vi "EI Example (B).vi"() -> ()   [LabVIEW 2011]
doc: "Electrochemical Interface control panel (basic version)."
uses:
  C:/Program Files/Metrohm Autolab/Autolab SDK 1.10/EcoChemie.Autolab.Sdk.dll
  EcoChemie.Autolab.Sdk.dll
panel:
  out "CurrentOverload":bool
  out "PotentialOverload":bool
  out "ManualCellSwitch":bool
  out "Cell":bool
  out "IsConnected":bool
  in  "stop":bool
  out "error out":errorcluster
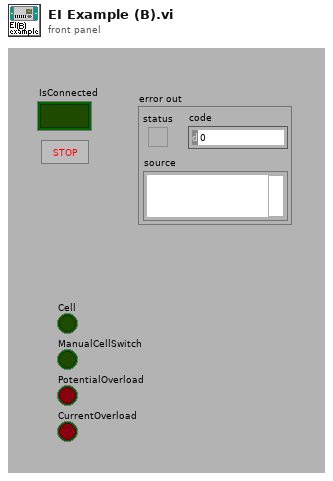
[diagram p1: front panel]
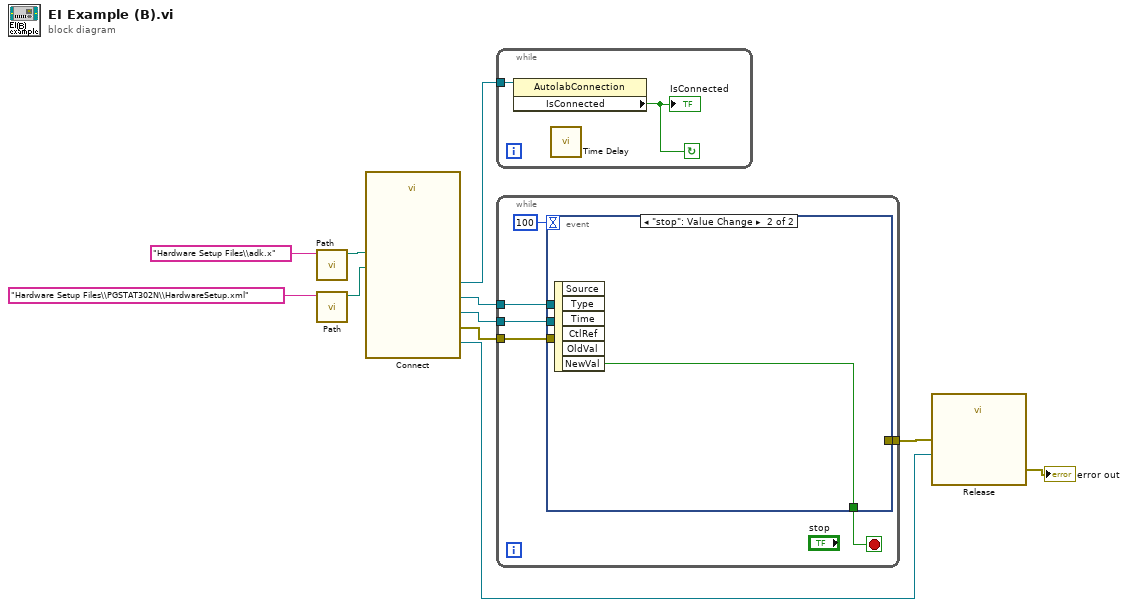
[diagram p0: block diagram]
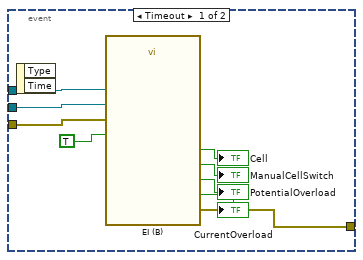
[diagram p2: hidden frame]
diagram:
  n1 = call "Path.vi"("name or relative path"="Hardware Setup Files\\adk.x") -> ("appended path"=w2:path)  [unwired: 10 in]
  n2 = call "Path.vi"("name or relative path"="Hardware Setup Files\\PGSTAT302N\\HardwareSetup.xml") -> ("appended path"=w1:path)  [unwired: 10 in]
  n3 = call "Connect.vi"("Embedded Exe File"=w2, "Hardware Setup File"=w1) -> ("Sampler"=w9:refnum<k24>, "AutolabConnection"=w11:refnum<k24>, "instrument"=w5:refnum<k24>, "Ei"=w10:refnum<k24>, "error out"=w8:errorcluster)  [unwired: 6 in, 3 out]
  n4 = while {
    tunnel: w11 -> [w12]
    stop <- w13 continue-if-true
    n5 = property class="AutolabConnection"(reference=w12) -> ("IsConnected"=w13:bool)  [unwired: 1 in, 2 out]
    "IsConnected" <- w13
    n6 = call "Time Delay"() -> ()  [unwired: 11 in, 1 out]
  }
  n7 = while {
    tunnel: [w16] -> w7
    tunnel: w10 -> [w19]
    tunnel: w9 -> [w18]
    tunnel: w8 -> [w17]
    stop <- w14 stop-if-true
    n8 = event shown="[1] \"stop\": Value Change" {
      selector: _ -> [_ _]
      dyn-events: _ -> [_ _]
      timeout: 100 -> [_ _]
      tunnel: w19 -> [w28 _]
      tunnel: w18 -> [w27 _]
      tunnel: w17 -> [w25 _]
      tunnel: [w20 _] -> w16
      tunnel: [_ w29] -> w14
      event Timeout {
        n9 = event-data() -> ()  [unwired: 1 in, 2 out]
        n10 = call "EI (B).vi"("Ei"=w28, "Sampler"=w27, "Disable Sampler"=TRUE, "error in (no error)"=w25) -> ("CurrentOverload"=→"CurrentOverload":bool, "PotentialOverload"=→"PotentialOverload":bool, "Cell"=→"Cell":bool, "ManualCellSwitch"=→"ManualCellSwitch":bool, "error out"=w20:errorcluster)  [unwired: 11 in]
      }
      event "stop": Value Change {
        n11 = event-data() -> ("NewVal"=w29:bool)  [unwired: 1 in, 5 out]
      }
    }
  }
  n12 = call "Release.vi"("error in (no error)"=w7, "Instrument"=w5) -> ("error out"=→"error out":errorcluster)  [unwired: 9 in]
